vi "gfitsio-read-key-logical.vi"(7 "keyname":string, 8 "error in (no error)":errorcluster, 9 "default value":bool, 11 "gfits refnum":T1) -> (0 "error out":errorcluster, 1 "comment":string, 2 "value":bool, 3 "dup gfits refnum":T1)   [LabVIEW 2019, in "gfitsio.lvlib"]
doc: "Return the specified keyword. <B>default value</B> specifies the desired returned data type of the keyword value. Data type conversion will be performed for numeric values if the keyword value does not have the same data type. If the keyword does not exist or an error occurs <B>value</B> will be equal to <B>default value</B>."
uses:
  gfitsio.lvlib
  gfitsio-refnum.ctl
  cfitsio-datatypes.ctl
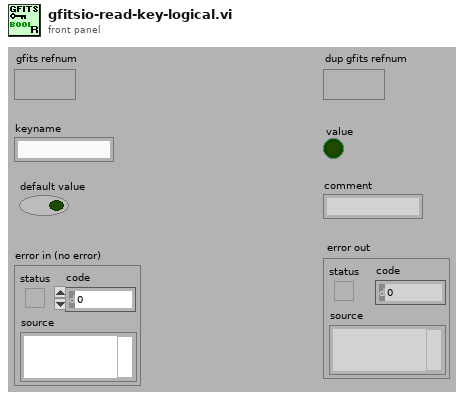
[diagram p1: front panel]
types:
  T1 = typedef "gfitsio.lvlib/gfitsio-refnum.ctl" = refnum<k1>
  T2 = typedef "gfitsio.lvlib/cfitsio-datatypes.ctl" = i32
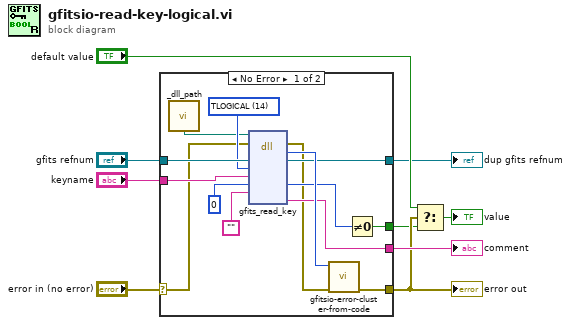
[diagram p0: block diagram]
diagram:
  n1 = case shown="No Error" "error in (no error)" {
    selector: "error in (no error)" -> [w12 w25]
    tunnel: [w22 w25] -> w3
    tunnel: "gfits refnum" -> [w20 w24]
    tunnel: [w21 w24] -> w1
    tunnel: "keyname" -> [w18 _]
    tunnel: [w13 _] -> w2
    tunnel: [w15 _] -> w4
    frame No Error {
      w19 = T2 14 items=["TBIT"=1, "TBYTE  (U8)"=11, "TSBYTE  (I8)"=12, "TLOGICAL"=14, "TSTRING"=16, "TUSHORT  (U16)"=20, "TSHORT  (I16)"=21, "TUINT"=31, "TULONG  (U32)"=40, "TLONG  (I32)"=41, "TFLOAT  (SGL)"=42, "TLONGLONG  (I64)"=81, "TDOUBLE  (DBL)"=82, "TCOMPLEX  (CSG)"=83, "TDOUBLECOMPLEX  (CDB)"=163] ("cfitsio datatype")
      n2 = call "_dll_path.vi"() -> ("Path"=w10:path)  [unwired: 1 in]
      n3 = dll-call lib="?" fn="gfits_read_key"(path in=w10, error in=w12, "refnum"=w20, "datatype"=w19, "keyname"=w18, "value"=u8 0, "units"="") -> (error out=w11:errorcluster, "return type"=w23:i32, "refnum"=w21:T1, "value"=w16:u8, "comment"=w15:string)  [unwired: 3 in, 3 out]
      n4 = call "gfitsio-error-cluster-from-code.vi"("error in (no error)"=w11, "error code"=w23) -> ("error out"=w22:errorcluster)  [unwired: 9 out]
      n5 = Not Equal To 0?(x=w16) -> (x != 0?=w13:bool)
    }
    frame Error {
    }
  }
  "error out" <- w3
  "dup gfits refnum" <- w1
  "comment" <- w4
  n6 = Select(t="default value", s=w3, f=w2) -> (s? t:f=→"value":bool)
